vi "Node Array to Diagram Clusters.vi"() -> ()   [LabVIEW 2024]
panel:
  in  "error in":errorcluster
  in  "Nodes[]":refnum<vi>[](array[refnum])
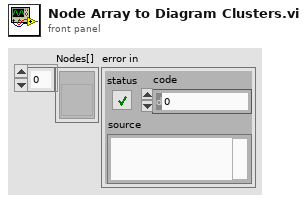
[diagram p1: front panel]
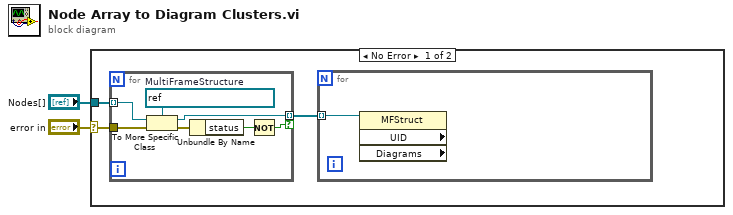
[diagram p0: block diagram]
diagram:
  n1 = case shown="No Error" "error in" {
    selector: "error in" -> [w4 _]
    tunnel: "Nodes[]" -> [w5 _]
    frame No Error {
      n2 = for {
        tunnel: w5 -> [w12] mode=indexing
        tunnel: w4 -> [w11]
        tunnel: [w10] -> w3 mode=indexing if=w7
        w13 = refnum<vi> refnum  # MultiFrameStructure
        n3 = To More Specific Class(target class=w13, reference=w12, error in=w11) -> (specific class reference=w10:refnum<vi>, error out=w9:errorcluster)
        n4 = Unbundle By Name(w9) -> ("status"=w8:bool)
        n5 = Not(x=w8) -> (.not. x?=w7:bool)
      }
      n6 = for {
        tunnel: w3 -> [w6] mode=indexing
        n7 = property class="MFStruct" props=["UID", "Diagrams"](reference=w6) -> ()  [unwired: 1 in, 4 out]
      }
    }
    frame Error {
    }
  }
